vi "Wait for Operation Complete.vi"(8 "error in (no error)":errorcluster, 10 "Timeout (10000 ms)":u32=10000, 11 "VISA resource name":refnum<visa-resource-name>) -> (0 "error out":errorcluster, 3 "VISA resource name out":refnum<visa-resource-name>)   [LabVIEW 2025, in "Keithley 2450.lvlib"]
doc: "Waits for an operation to complete. This is useful for synchronizing instrument code with other code.\n\n<B>Note:</B> When taking measurements, this VI will hold until the instrument has armed and triggered all of the times specified in Configure Multipoint. This VI won't function correctly if the triggering has occured but the instrument is set to arm after those triggered measurements have finished.\n\nUse this VI only with other low-level VIs. The high-level VIs automatically incorporate this functionality. This VI does not check the instrument status. If you want to check the instrument status, call the Error Query VI at the conclusion of the sequence."
uses:
  Keithley 2450.lvlib
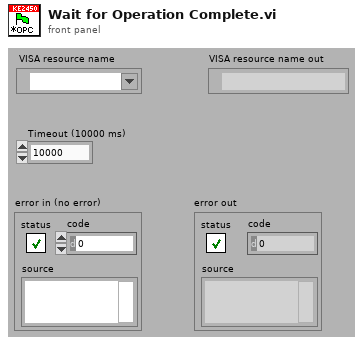
[diagram p1: front panel]
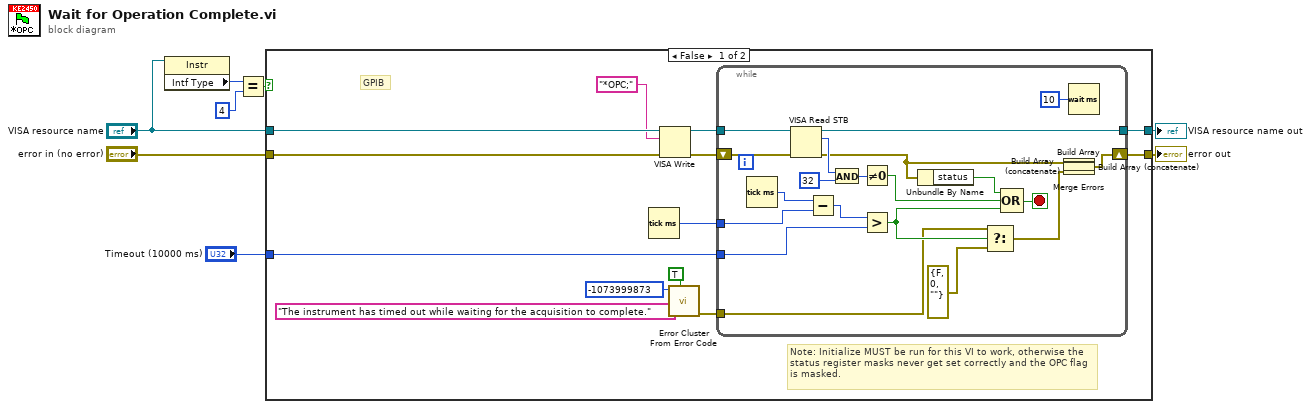
[diagram p0: block diagram]
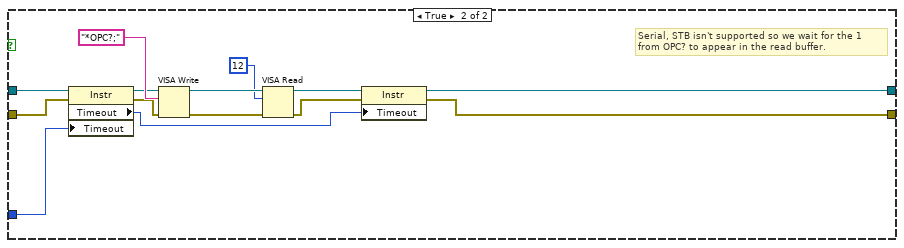
[diagram p2: hidden frame]
diagram:
  n1 = property class="Instr"(reference="VISA resource name") -> ("Intf Type"=w3:u16)  [unwired: 1 in, 2 out]
  n2 = Equal?(x=w3, y=u16 4) -> (x = y?=w4:bool)
  n3 = case shown="False" w4 {
    tunnel: "VISA resource name" -> [w21 w54]
    tunnel: "error in (no error)" -> [w20 w49]
    tunnel: [w17 w45] -> w7
    tunnel: [w16 w50] -> w6
    tunnel: "Timeout (10000 ms)" -> [w9 w53]
    frame False {
      # "GPIB"
      # "Note: Initialize MUST be run for this VI to work, otherwise the status register masks never get set correctly and the OPC flag is masked."
      n4 = Tick Count (ms)() -> (millisecond timer value=w14:u32)
      n5 = VISA Write(VISA resource name=w21, write buffer="*OPC;", error in (no error)=w20) -> (VISA resource name out=w19:refnum<visa-resource-name>, error out=w18:errorcluster)  [unwired: 1 out]
      n6 = call <vilib>:"Error Cluster From Error Code.vi"("show call chain? (False)"=TRUE, "error message (\"\")"="The instrument has timed out while waiting for the acquisition to complete." ("error message (\"\")"), "error code (0)"=-1073999873) -> ("error out"=w10:errorcluster)  [unwired: 1 in, 5 out]
      n7 = while {
        tunnel: w19 -> [w44]
        tunnel: [w42] -> w16
        tunnel: w14 -> [w37]
        shift-right: [w29] -> w17
        shift-left: w18 -> [w43]
        tunnel: w10 -> [w32]
        tunnel: w9 -> [w25]
        stop <- w34 stop-if-true
        n8 = Tick Count (ms)() -> (millisecond timer value=w38:u32)
        n9 = VISA Read STB(8:w43, 11:w44) -> (0:w28:errorcluster, 2:w41:u16, 3:w42:refnum<visa-resource-name>)
        n10 = Subtract(x=w38, y=w37) -> (x-y=w36:u32)
        n11 = And(x=w41, y=u16 32) -> (x .and. y?=w39:u16)
        n12 = Not Equal To 0?(x=w39) -> (x != 0?=w35:bool)
        n13 = Greater?(x=w36, y=w25) -> (0:w33:bool)
        n14 = Unbundle By Name(w28) -> ("status"=w27:bool)
        n15 = Select(t=w32, s=w33, f=errorcluster {"status"=FALSE, "code"=0, "source"=""}) -> (s? t:f=w30:errorcluster)
        n16 = Compound Arithmetic op=OR(w27, w35, w33) -> (w34:bool)
        n17 = Build Array(w28, w30) -> (w24:errorcluster[])
        n18 = Build Array (concatenate)(w24) -> (w23:errorcluster[])
        n19 = Build Array (concatenate)(w23) -> (w22:errorcluster[])
        n20 = Merge Errors(w22) -> (w29:errorcluster)
        n21 = Wait (ms)(milliseconds to wait=u32 10) -> ()  [unwired: 1 out]
      }
    }
    frame True {
      # "Serial, STB isn't supported so we wait for the 1 \nfrom OPC? to appear in the read buffer."
      n22 = property class="Instr"(reference=w54, error in=w49, "Timeout"=w53) -> (reference out=w48:refnum<visa-resource-name>, error out=w47:errorcluster, "Timeout"=w52:u32)
      n23 = VISA Write(VISA resource name=w48, write buffer="*OPC?;", error in (no error)=w47) -> (VISA resource name out=w56:refnum<visa-resource-name>, error out=w57:errorcluster)  [unwired: 1 out]
      n24 = VISA Read(VISA resource name=w56, byte count=u32 12, error in (no error)=w57) -> (VISA resource name out=w51:refnum<visa-resource-name>, error out=w46:errorcluster)  [unwired: 2 out]
      n25 = property class="Instr"(reference=w51, error in=w46, "Timeout"=w52) -> (reference out=w50:refnum<visa-resource-name>, error out=w45:errorcluster)
    }
  }
  "VISA resource name out" <- w6
  "error out" <- w7
